vi "TestExec.Record Installation Update to File.vi"(9 "Version":string, 10 "Name":string, 11 "AppDataDir":path) -> (3 "Initial Install":bool)   [LabVIEW 2019]
uses:
  <vilib>/KATE/Files/File Utils.lvlib
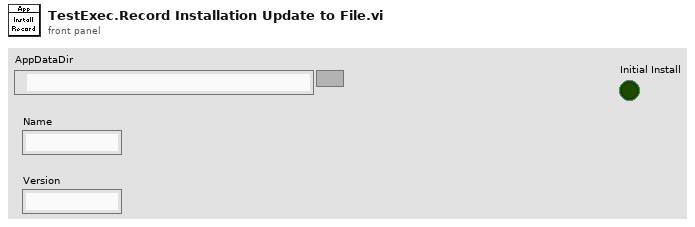
[diagram p1: front panel]
types:
  T1 = enum16{"open", "replace", "create", "open or create", "replace or create", "replace or create with confirmation"}
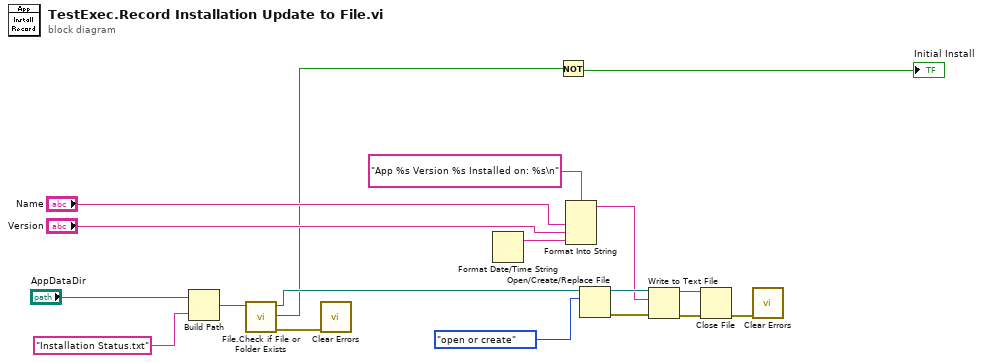
[diagram p0: block diagram]
diagram:
  n1 = Build Path(base path="AppDataDir", name or relative path="Installation Status.txt") -> (appended path=w14:path)
  n2 = call <vilib>:"File.Check if File or Folder Exists.vi"("Path"=w14) -> ("error out"=w1:errorcluster, "Exists"=w12:bool, "Dup Path"=w13:path)  [unwired: 6 in, 2 out]
  n3 = call <vilib>:"Clear Errors.vi"("error in (no error)"=w1) -> ()  [unwired: 5 in, 2 out]
  n4 = Format Date/Time String() -> (date/time string=w2:string)  [unwired: 3 in]
  n5 = Not(x=w12) -> (.not. x?=→"Initial Install":bool)
  n6 = Format Into String(format string="App %s Version %s Installed on: %s\n" ("name or relative path"), "Name", "Version", w2) -> (resulting string=w3:string)  [unwired: 2 in, 1 out]
  n7 = Open/Create/Replace File(file path (use dialog)=w13, operation (0:open)=T1."open or create") -> (refnum out=w7:refnum<file>, error out=w6:errorcluster)  [unwired: 4 in, 1 out]
  n8 = Write to Text File(file (use dialog)=w7, text=w3, error in=w6) -> (refnum out=w9:refnum<file>, error out=w10:errorcluster)  [unwired: 1 in, 1 out]
  n9 = Close File(refnum=w9, error in=w10) -> (error out=w8:errorcluster)  [unwired: 1 out]
  n10 = call <vilib>:"Clear Errors.vi"("error in (no error)"=w8) -> ()  [unwired: 5 in, 2 out]
